vi "Do.vi"(8 "error in (no error)":errorcluster, 10 "Actor in":refnum<class "Actor.lvclass">, 11 "Test Progress Msg":refnum<class "Test Progress Msg.lvclass">) -> (0 "error out":errorcluster, 2 "Actor out":refnum<class "Actor.lvclass">)   [LabVIEW 2017, in "Test Application Controller.lvlib" / "Test Progress Msg.lvclass"]
doc: "This VI delivers the message to the actor by calling the appropriate method(s) on the actor."
uses:
  Test Progress Msg.lvclass
  D:/Career/Tesla/LabVIEW_Interview_Problem/Tesla Test Application/Test/Test Messages/Test Progress Msg/Test Progress Msg.lvclass
  <vilib>/ActorFramework/Actor/Actor.lvclass
  Test Application Controller/Test Application Controller.lvclass
  C:/Program Files (x86)/National Instruments/LabVIEW 2017/vi.lib/ActorFramework/Actor/Actor.lvclass
  Test/Test Messages/Test Progress Msg/Test Progress Msg.lvclass/Test Progress Msg.ctl
  Test/Test Messages/Test Progress Msg/Test Progress Msg.lvclass
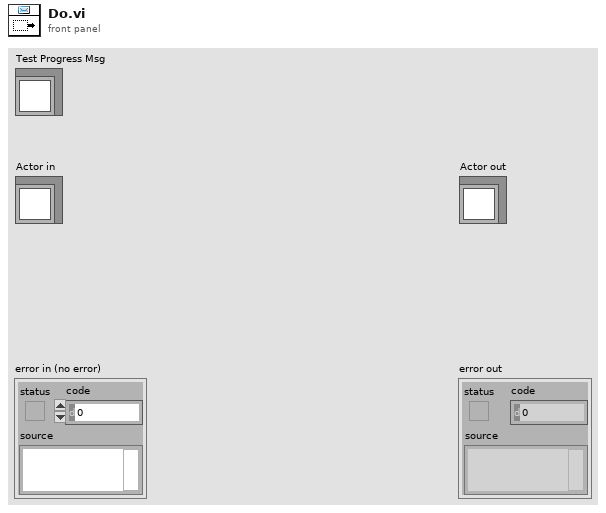
[diagram p1: front panel]
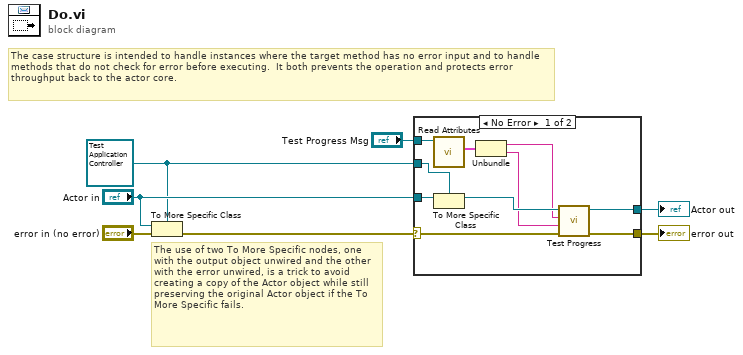
[diagram p0: block diagram]
diagram:
  w2 = refnum<class "Test Application Controller.lvclass"> refnum ("Actor in")
  # "The use of two To More Specific nodes, one with the output object unwired and the other with the error unwired, is a trick to avoid creating a copy of the Actor object while still preserving the original Actor object if the To More Specific fails."
  # "The case structure is intended to handle instances where the target method has no error input and to handle methods that do not check for error before executing.  It both prevents the operation and protects error throughput back to the actor core."
  n1 = To More Specific Class(target class=w2, reference="Actor in", error in="error in (no error)") -> (error out=w6:errorcluster)  [unwired: 1 out]
  n2 = case shown="No Error" w6 {
    selector: w6 -> [w15 w19]
    tunnel: [w17 w19] -> w5
    tunnel: [w16 w18] -> w4
    tunnel: "Actor in" -> [w14 w18]
    tunnel: w2 -> [w13 _]
    tunnel: "Test Progress Msg" -> [w10 _]
    frame No Error {
      n3 = call "Read Attributes.vi"("Test Progress Msg"=w10) -> ("Payload"=w11:cluster{"Test Name":string, "State":string})  [unwired: 10 in]
      n4 = To More Specific Class(target class=w13, reference=w14) -> (specific class reference=w12:refnum<class "Test Application Controller.lvclass">)  [unwired: 1 in, 1 out]
      n5 = Unbundle(w11) -> ("Test Name"=w9:string, "State"=w8:string)
      n6 = call "Test Progress.vi"("error in (no error)"=w15, "Current State"=w8, "Test Name"=w9, "Test Application Controller in"=w12) -> ("error out"=w17:errorcluster, "Test Application Controller out"=w16:refnum<class "Test Application Controller.lvclass">)  [unwired: 6 in]
    }
    frame Error {
      # "If type check fails, pass the original object out again."
    }
  }
  "error out" <- w5
  "Actor out" <- w4
